vi "gesture.vi"() -> ()   [LabVIEW 2012]
uses:
  <vilib>/University of Leeds/Kinesthesia Toolkit for Microsoft Kinect/_Polymorphic Configure/Event-Skeleton.vi
  <vilib>/University of Leeds/Kinesthesia Toolkit for Microsoft Kinect/_Polymorphic Close/Close-Skeleton.vi
  <vilib>/University of Leeds/Kinesthesia Toolkit for Microsoft Kinect/_Polymorphic Read/Read-Skeleton.vi
panel:
  in  "文件路径（使用对话框）":path=path "E:/djangowork/ni/main/status.txt"
  out "连接的字符串":string
  in  "Target":string="dstp://localhost/para" caption="目标"
  out "量表":dbl(knob) scale=-180.0..180.0
  out "转动状态标识":u8
  out "待转度数":dbl
  out "state":u8
  out "缩放手势识别":bool
  out "放大杆":dbl(slide) scale=0.5..1000.0
  in  "左手z数组":dbl[](array[numeric])
  in  "右手z数组":dbl[](array[numeric])
  out "缩放手势计数":u8
  in  "下限":dbl
  in  "上限":dbl=0.2
  in  "左肩y数组":dbl[](array[numeric])
  in  "右手y数组":dbl[](array[numeric])
  in  "右划阈值":dbl=0.08
  in  "左划阈值":dbl=-0.08
  in  "右上下阈值":dbl=0.2
  out "右挥手势判断":bool
  in  "左上下阈值":dbl=0.2
  in  "右手x数组":dbl[](array[numeric])
  in  "左手y数组":dbl[](array[numeric])
  out "左挥手势判断":bool
  in  "数组索引":i32
  in  "左手x数组":dbl[](array[numeric])
  in  "布尔":bool
  out "error out":errorcluster
  in  "error in (no error)":errorcluster
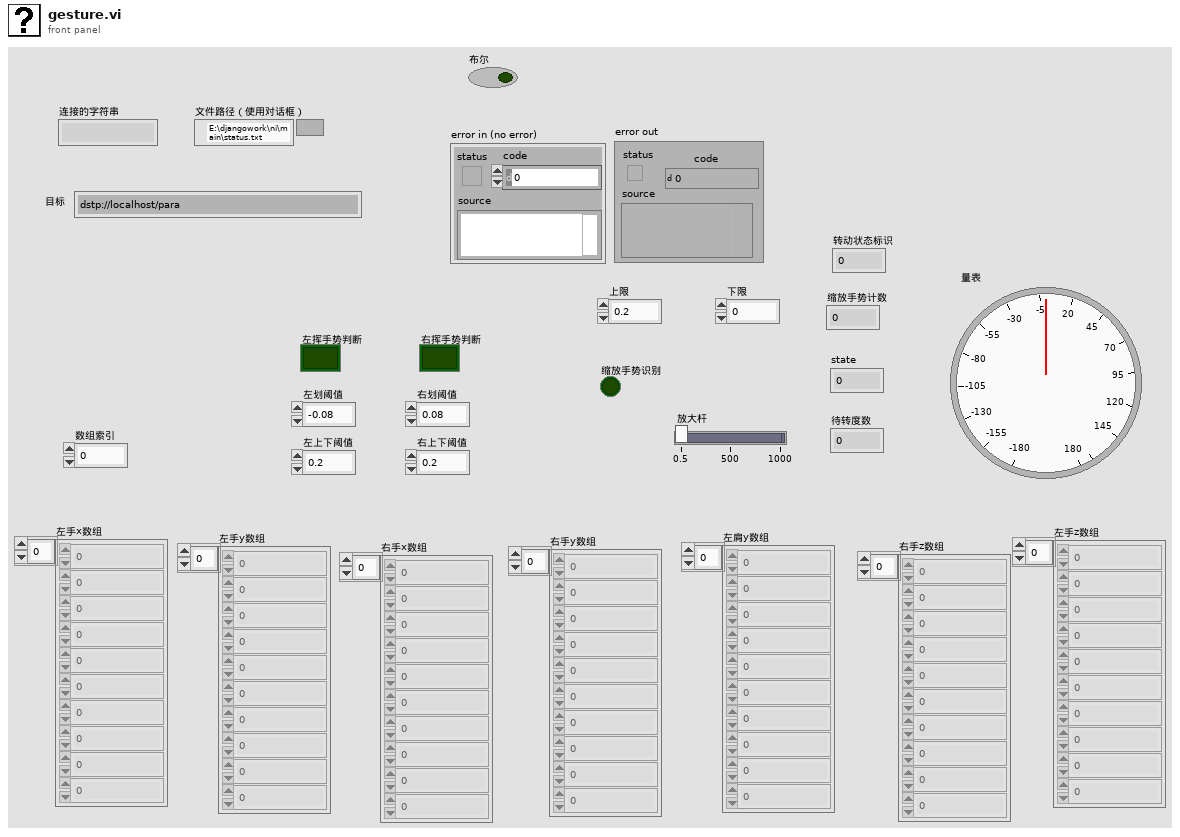
[diagram p1: front panel]
types:
  T1 = cluster{cluster{"reference out":refnum<k24>, "KinectSensors":refnum<k24>}, "get_Item":refnum<k24>}
  T2 = cluster{"reference out":refnum<k24>, "KinectSensors":refnum<k24>, "SkeletonStream":refnum<k24>, refnum<k24>[], "get_Item":refnum<k24>}
  T3 = enum16{"hip centre", "spine", "shoulder centre", "head", "shoulder left", "elbow left", "wrist left", "hand left", "shoulder right", "elbow right", "wrist right", "hand right", "hip left", "knee left", "ankle left", "foot left", "hip right", "knee right", "ankle right", "foot right"}
  T4 = enum16{"open", "replace", "create", "open or create", "replace or create", "replace or create with confirmation"}
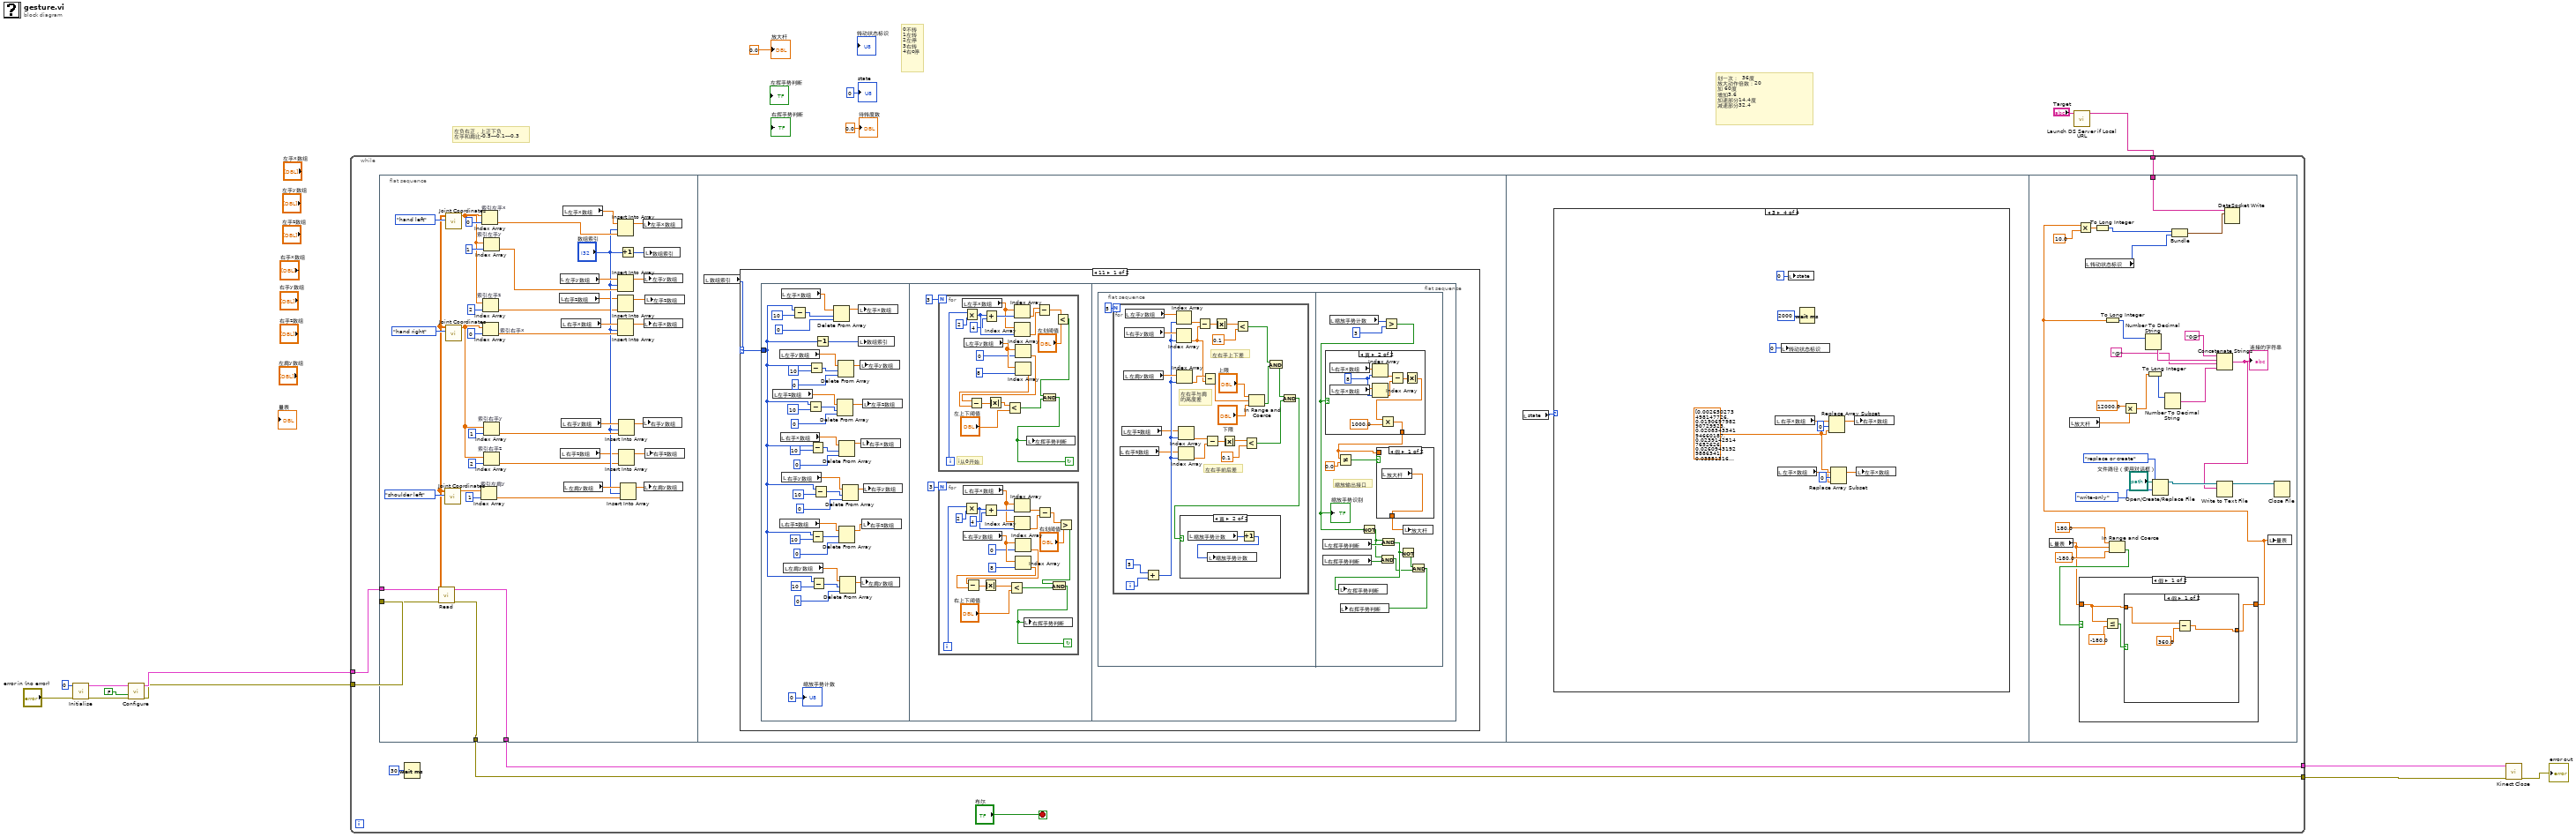
[diagram p0: block diagram]
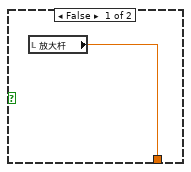
[diagram p4: hidden frame]
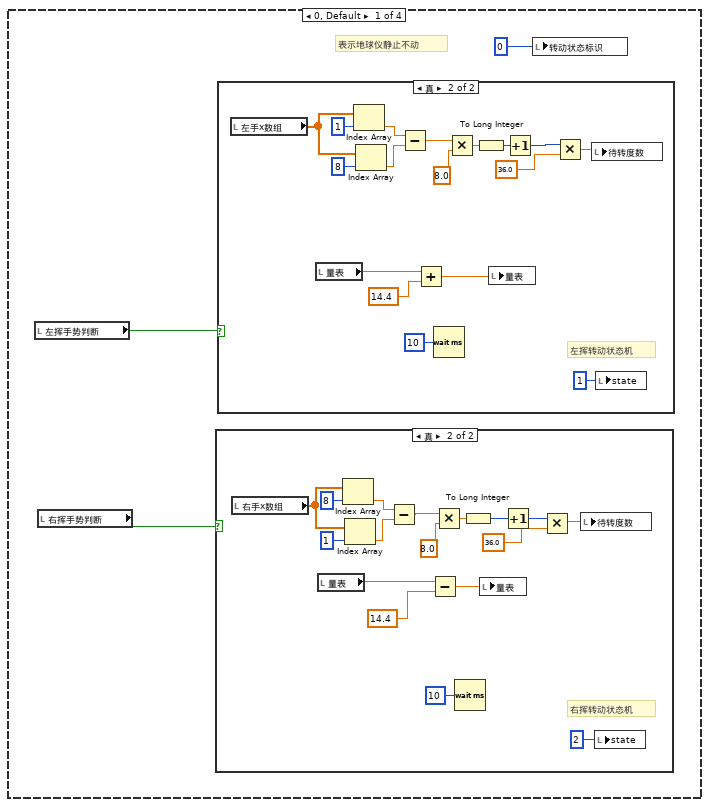
[diagram p6: hidden frame]
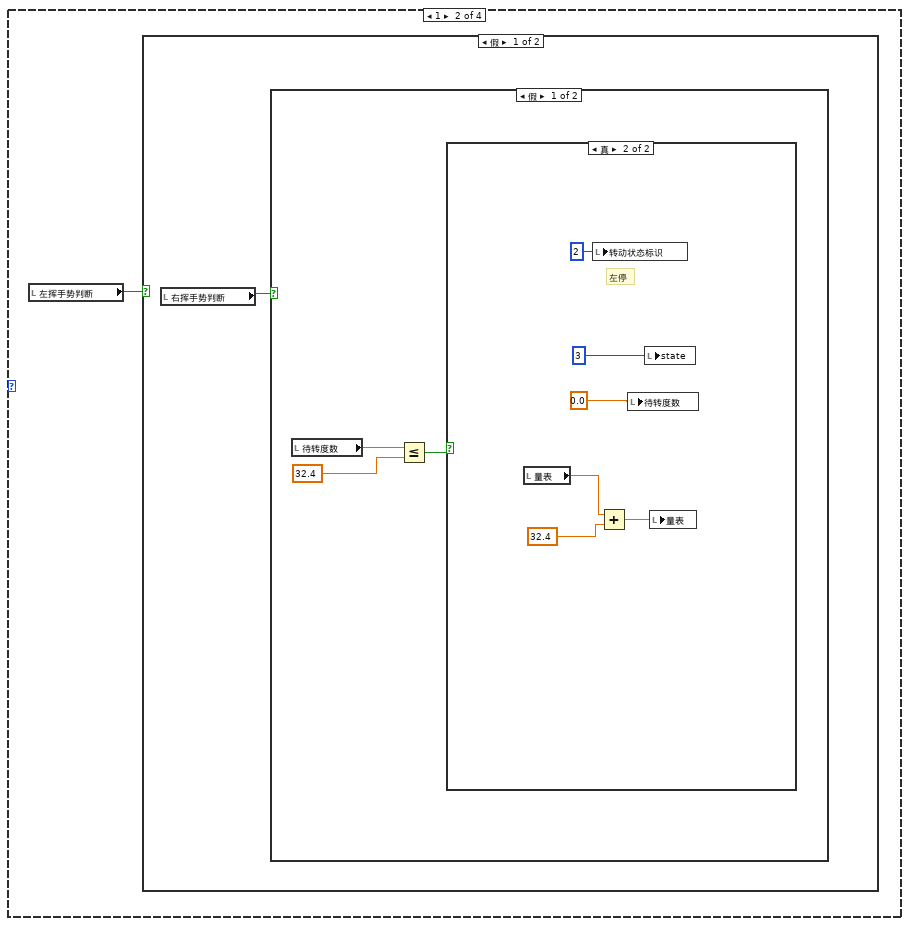
[diagram p9: hidden frame]
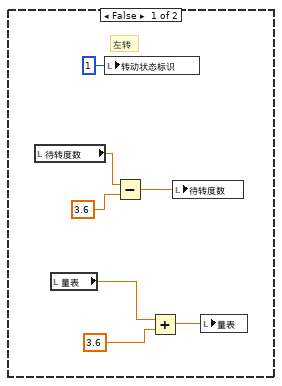
[diagram p10: hidden frame]
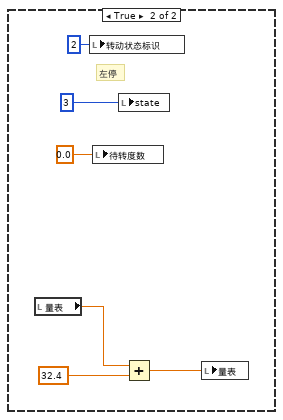
[diagram p11: hidden frame]
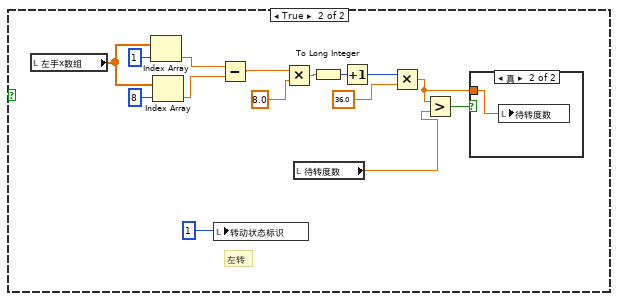
[diagram p12: hidden frame]
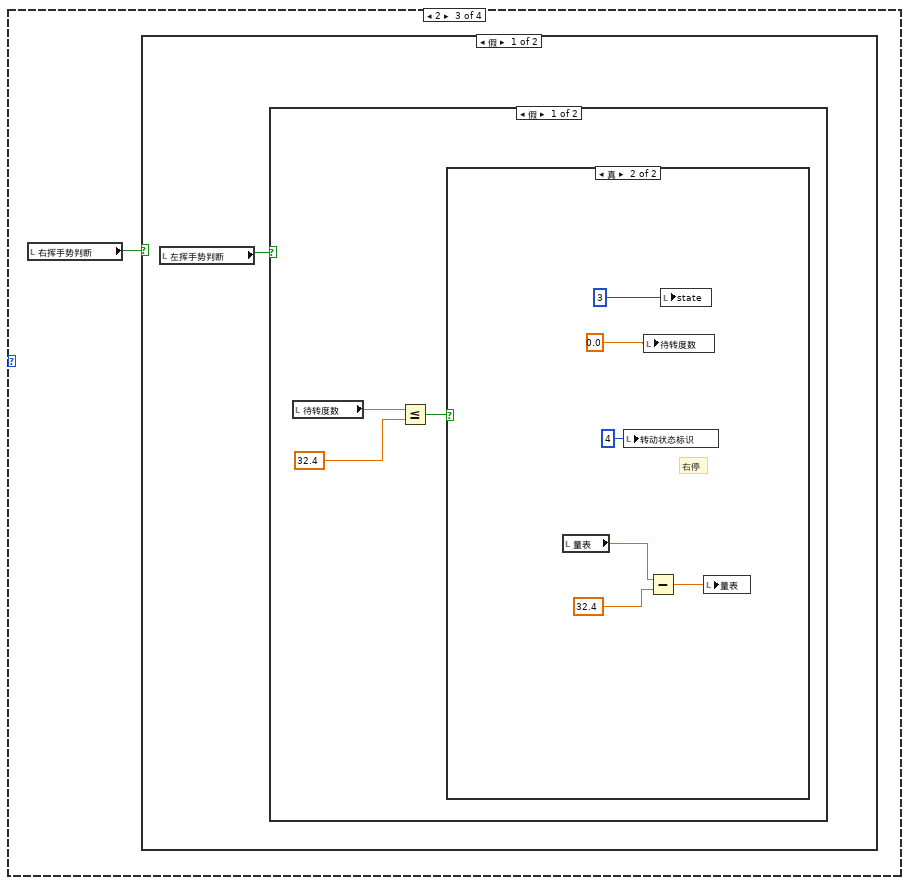
[diagram p14: hidden frame]
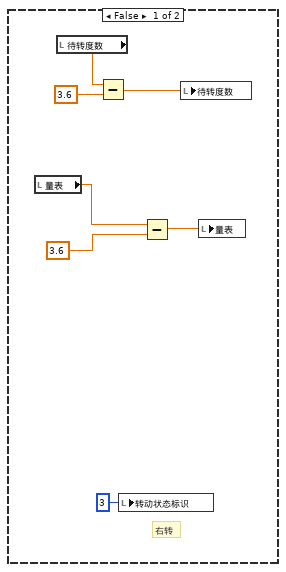
[diagram p15: hidden frame]
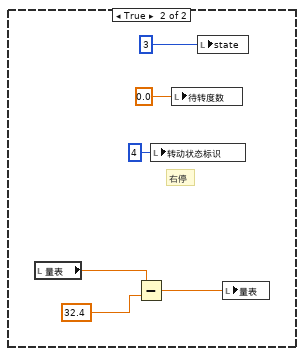
[diagram p16: hidden frame]
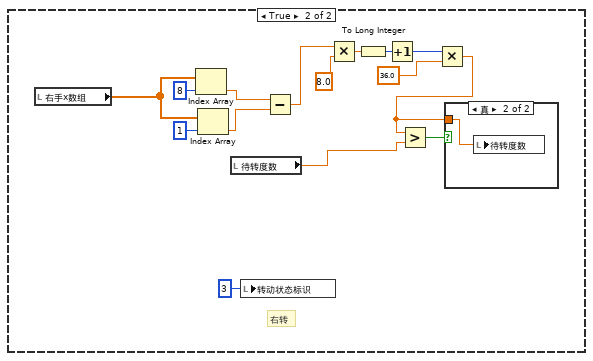
[diagram p17: hidden frame]
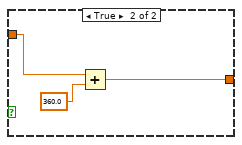
[diagram p19: hidden frame]
diagram:
  # "划一次：  36度\n放大动作倍数：20\n加 60度\n增加3.6\n加速部分14.4度\n减速部分32.4"
  # "0不转\n1左转\n2左停\n3右转\n4右c停"
  # "左负右正，上正下负\n左手和肩比-0.5---0.1---0.3"
  n1 = call <vilib>:"Initialise.vi"("Kinect Number"=0, "error in (no error)"="error in (no error)") -> ("Kinect References out"=w11:T1, "error out"=w14:errorcluster)  [unwired: 12 in]
  n2 = call-poly <vilib>:"Configure.vi"("Kinect References in"=w11, "Skeleton Smoothing"=FALSE, "error in"=w14) -> ("Kinect References out"=w10:T2, "error out"=w9:errorcluster)  [unwired: 11 in]
  n3 = call <vilib>:"Launch DS Server if Local URL.vi"("URL"="Target") -> ("Duplicate URL"=w2:string)  [unwired: 1 in, 5 out]
  n4 = while {
    tunnel: w10 -> [w20]
    tunnel: w9 -> [w21]
    tunnel: [w19] -> w8
    tunnel: [w18] -> w7
    tunnel: w2 -> [w16]
    stop <- "布尔" stop-if-true
    n5 = flat-sequence {
      tunnel: w21 -> [w63]
      tunnel: w20 -> [w62]
      tunnel: [w61] -> w19
      tunnel: [w60] -> w18
      tunnel: w16 -> [w339]
      frame #0 {
        n6 = call-poly <vilib>:"Read.vi"("Kinect References in"=w62, "error in (no error)"=w63) -> ("Primary Skeleton Array"=w37:dbl[][], "Kinect References out"=w61:T2, "error out"=w60:errorcluster)  [unwired: 10 in, 1 out]
        n7 = call <vilib>:"Joint Coordinates.vi"("Joint 1"=T3."shoulder left", "Array of Joint Positions"=w37) -> ("Joint Coordinates"=w38:dbl[])  [unwired: 8 in, 1 out]
        n8 = call <vilib>:"Joint Coordinates.vi"("Joint 1"=T3."hand left", "Array of Joint Positions"=w37) -> ("Joint Coordinates"=w28:dbl[])  [unwired: 8 in, 1 out]
        n9 = call <vilib>:"Joint Coordinates.vi"("Joint 1"=T3."hand right", "Array of Joint Positions"=w37) -> ("Joint Coordinates"=w27:dbl[])  [unwired: 8 in, 1 out]
        n10 = Index Array "索引左肩y"(array=w38, index=1 ("索引")) -> (element=w36:dbl)
        n11 = Index Array "索引左手x"(array=w28, index=0 ("索引")) -> (element=w56:dbl)
        n12 = Index Array "索引左手z"(array=w28, index=2 ("索引")) -> (element=w29:dbl)
        n13 = Index Array "索引右手x"(array=w27, index=0 ("索引")) -> (element=w47:dbl)
        n14 = Index Array "索引左手y"(array=w28, index=1 ("索引")) -> (element=w52:dbl)
        n15 = Index Array "索引右手y"(array=w27, index=1 ("索引")) -> (element=w43:dbl)
        n16 = Index Array "索引右手z"(array=w27, index=2 ("索引")) -> (element=w31:dbl)
        n17 = local read "右手z数组"() -> (w26:dbl[])
        n18 = local read "左手y数组"() -> (w51:dbl[])
        n19 = local read "右手z数组"() -> (w23:dbl[])
        n20 = local read "右手x数组"() -> (w46:dbl[])
        n21 = local read "右手y数组"() -> (w41:dbl[])
        n22 = local read "左手x数组"() -> (w55:dbl[])
        n23 = local read "左肩y数组"() -> (w35:dbl[])
        n24 = Insert Into Array(array=w55, index="数组索引", new element=w56) -> (w54:dbl[])
        n25 = Insert Into Array(array=w51, index="数组索引", new element=w52) -> (w50:dbl[])
        n26 = Insert Into Array(array=w26, new element=w29) -> (w25:dbl[])  [unwired: 1 in]
        n27 = Insert Into Array(array=w46, index="数组索引", new element=w47) -> (w45:dbl[])
        n28 = Insert Into Array(array=w41, index="数组索引", new element=w43) -> (w42:dbl[])
        n29 = Insert Into Array(array=w23, new element=w31) -> (w24:dbl[])  [unwired: 1 in]
        n30 = Increment(x="数组索引") -> (x+1=w53:i32)
        n31 = Insert Into Array(array=w35, index="数组索引", new element=w36) -> (w34:dbl[])
        n32 = local write "左手x数组"(w54) -> ()
        n33 = local write "右手y数组"(w42) -> ()
        n34 = local write "左手y数组"(w50) -> ()
        n35 = local write "右手x数组"(w45) -> ()
        n36 = local write "左肩y数组"(w34) -> ()
        n37 = local write "数组索引"(w53) -> ()
        n38 = local write "右手z数组"(w24) -> ()
        n39 = local write "左手z数组"(w25) -> ()
      }
      frame #1 {
        n40 = local read "数组索引"() -> (w64:i32)
        n41 = case shown="11" w64 {
          selector: w64 -> [w65 _]
          frame 11 {
            n42 = flat-sequence {
              tunnel: w65 -> [w66]
              frame #0 {
                n43 = local read "左手z数组"() -> (w70:dbl[])
                n44 = local read "左手y数组"() -> (w91:dbl[])
                n45 = local read "右手z数组"() -> (w67:dbl[])
                n46 = local read "右手x数组"() -> (w90:dbl[])
                n47 = local read "左手x数组"() -> (w102:dbl[])
                n48 = local read "右手y数组"() -> (w84:dbl[])
                n49 = local read "左肩y数组"() -> (w79:dbl[])
                n50 = Subtract(x=w66, y=10) -> (x-y=w99:i32)
                n51 = Subtract(x=w66, y=10) -> (x-y=w72:i32)
                n52 = Subtract(x=w66, y=10) -> (x-y=w95:i32)
                n53 = Subtract(x=w66, y=10) -> (x-y=w92:i32)
                n54 = Subtract(x=w66, y=10) -> (x-y=w75:i32)
                n55 = Subtract(x=w66, y=10) -> (x-y=w81:i32)
                n56 = Subtract(x=w66, y=10) -> (x-y=w86:i32)
                n57 = Decrement(x=w66) -> (x-1=w98:i32)
                n58 = Delete From Array(array=w102, length=w99, index=0 ("索引")) -> (array with subset deleted=w101:dbl[])  [unwired: 1 out]
                n59 = Delete From Array(array=w70, length=w72, index=0 ("索引")) -> (array with subset deleted=w69:dbl[])  [unwired: 1 out]
                n60 = Delete From Array(array=w91, length=w95, index=0 ("索引")) -> (array with subset deleted=w89:dbl[])  [unwired: 1 out]
                n61 = Delete From Array(array=w90, length=w92, index=0 ("索引")) -> (array with subset deleted=w88:dbl[])  [unwired: 1 out]
                n62 = Delete From Array(array=w67, length=w75, index=0 ("索引")) -> (array with subset deleted=w68:dbl[])  [unwired: 1 out]
                n63 = Delete From Array(array=w79, length=w81, index=0 ("索引")) -> (array with subset deleted=w78:dbl[])  [unwired: 1 out]
                n64 = Delete From Array(array=w84, length=w86, index=0 ("索引")) -> (array with subset deleted=w83:dbl[])  [unwired: 1 out]
                n65 = local write "左手x数组"(w101) -> ()
                n66 = local write "数组索引"(w98) -> ()
                n67 = local write "左手y数组"(w89) -> ()
                n68 = local write "左肩y数组"(w78) -> ()
                n69 = local write "右手x数组"(w88) -> ()
                n70 = local write "右手z数组"(w68) -> ()
                n71 = local write "左手z数组"(w69) -> ()
                n72 = local write "右手y数组"(w83) -> ()
                "缩放手势计数" <- u8 0 ("放大判断计数")
              }
              frame #1 {
                n73 = for {
                  N: 3 -> [_]
                  i -> [w142]
                  stop <- w134 continue-if-true
                  # "i从0开始"
                  n74 = local read "左手x数组"() -> (w145:dbl[])
                  n75 = local read "左手y数组"() -> (w133:dbl[])
                  n76 = Multiply(x=w142, y=2) -> (x*y=w144:i32)
                  n77 = Add(x=w144, y=4) -> (x+y=w146:i32)
                  n78 = Index Array(array=w145, index=w146) -> (element=w132:dbl)
                  n79 = Index Array(array=w145, index=w144) -> (element=w131:dbl)
                  n80 = Index Array(array=w133, index=0 ("索引")) -> (element=w141:dbl)
                  n81 = Index Array(array=w133, index=8 ("索引")) -> (element=w140:dbl)
                  n82 = Subtract(x=w141, y=w140) -> (x-y=w139:dbl)
                  n83 = Absolute Value(x=w139) -> (abs(x)=w138:dbl)
                  n84 = Less?(x=w138, y="左上下阈值") -> (x < y?=w135:bool)
                  n85 = Subtract(x=w132, y=w131) -> (x-y=w130:dbl)
                  n86 = Less?(x=w130, y="左划阈值") -> (x < y?=w136:bool)
                  n87 = And(x=w136, y=w135) -> (x .and. y?=w134:bool)
                  n88 = local write "左挥手势判断"(w134) -> ()
                }
                n89 = for {
                  N: 3 -> [_]
                  i -> [w122]
                  stop <- w111 continue-if-true
                  n90 = local read "右手y数组"() -> (w120:dbl[])
                  n91 = local read "右手x数组"() -> (w121:dbl[])
                  n92 = Multiply(x=w122, y=2) -> (x*y=w123:i32)
                  n93 = Add(x=w123, y=4) -> (x+y=w124:i32)
                  n94 = Index Array(array=w121, index=w124) -> (element=w119:dbl)
                  n95 = Index Array(array=w121, index=w123) -> (element=w118:dbl)
                  n96 = Index Array(array=w120, index=0 ("索引")) -> (element=w117:dbl)
                  n97 = Index Array(array=w120, index=8 ("索引")) -> (element=w116:dbl)
                  n98 = Subtract(x=w117, y=w116) -> (x-y=w115:dbl)
                  n99 = Absolute Value(x=w115) -> (abs(x)=w113:dbl)
                  n100 = Less?(x=w113, y="右上下阈值") -> (x < y?=w112:bool)
                  n101 = Subtract(x=w119, y=w118) -> (x-y=w110:dbl)
                  n102 = Greater?(x=w110, y="右划阈值") -> (0:w109:bool)
                  n103 = And(x=w109, y=w112) -> (x .and. y?=w111:bool)
                  n104 = local write "右挥手势判断"(w111) -> ()
                }
              }
              frame #2 {
                n105 = flat-sequence {
                  frame #0 {
                    n106 = for {
                      N: 5 -> [_]
                      i -> [w161]
                      # "左右手上下差"
                      # "左右手前后差"
                      # "左右手与肩\n的高度差"
                      n107 = local read "右手z数组"() -> (w157:dbl[])
                      n108 = local read "左手z数组"() -> (w158:dbl[])
                      n109 = local read "左肩y数组"() -> (w170:dbl[])
                      n110 = local read "右手y数组"() -> (w174:dbl[])
                      n111 = local read "左手y数组"() -> (w175:dbl[])
                      n112 = Add(x=5, y=w161) -> (x+y=w159:i32)
                      n113 = Index Array(array=w175, index=w159) -> (element=w173:dbl)
                      n114 = Index Array(array=w174, index=w159) -> (element=w168:dbl)
                      n115 = Index Array(array=w170, index=w159) -> (element=w169:dbl)
                      n116 = Index Array(array=w158, index=w159) -> (element=w155:dbl)
                      n117 = Index Array(array=w157, index=w159) -> (element=w154:dbl)
                      n118 = Subtract(x=w173, y=w168) -> (x-y=w162:dbl)
                      n119 = Subtract(x=w169, y=w168) -> (x-y=w165:dbl)
                      n120 = Subtract(x=w155, y=w154) -> (x-y=w156:dbl)
                      n121 = Absolute Value(x=w162) -> (abs(x)=w172:dbl)
                      n122 = Absolute Value(x=w156) -> (abs(x)=w153:dbl)
                      n123 = Less?(x=w172, y=0.1 ("左右手上下差")) -> (x < y?=w163:bool)
                      n124 = Less?(x=w153, y=0.1 ("左右手前后差")) -> (x < y?=w151:bool)
                      n125 = In Range and Coerce(upper limit="上限", x=w165, lower limit="下限") -> (In Range?=w164:bool)  [unwired: 1 out]
                      n126 = And(x=w163, y=w164) -> (x .and. y?=w152:bool)
                      n127 = And(x=w152, y=w151) -> (x .and. y?=w150:bool)
                      n128 = case shown="真" w150 {
                        frame False {
                        }
                        frame True {
                          n129 = local read "缩放手势计数"() -> (w177:u8)
                          n130 = Increment(x=w177) -> (x+1=w176:u8)
                          n131 = local write "缩放手势计数"(w176) -> ()
                        }
                      }
                    }
                  }
                  frame #1 {
                    # "缩放输出接口"
                    n132 = local read "左挥手势判断"() -> (w188:bool)
                    n133 = local read "右挥手势判断"() -> (w186:bool)
                    n134 = local read "缩放手势计数"() -> (w191:u8)
                    n135 = Greater?(x=w191, y=u8 3) -> (0:w182:bool)
                    "缩放手势识别" <- w182
                    n136 = case shown="真" w182 {
                      tunnel: [w194 w197] -> w179
                      frame False {
                        n137 = local read "放大杆"() -> (w194:dbl)
                      }
                      frame True {
                        w195 = 8 ("索引")
                        n138 = local read "右手x数组"() -> (w202:dbl[])
                        n139 = local read "左手x数组"() -> (w203:dbl[])
                        n140 = Index Array(array=w202, index=w195) -> (element=w200:dbl)
                        n141 = Index Array(array=w203, index=w195) -> (element=w199:dbl)
                        n142 = Subtract(x=w200, y=w199) -> (x-y=w201:dbl)
                        n143 = Absolute Value(x=w201) -> (abs(x)=w198:dbl)
                        n144 = Multiply(x=w198, y=1000.0 ("调整")) -> (x*y=w197:dbl)
                      }
                    }
                    n145 = Not Equal?(x=w179, y=0.0) -> (x != y?=w181:bool)
                    n146 = Not(x=w182) -> (.not. x?=w187:bool)
                    n147 = case shown="假" w181 {
                      tunnel: w179 -> [_ w193]
                      tunnel: [w192 w193] -> w178
                      frame False {
                        n148 = local read "放大杆"() -> (w192:dbl)
                      }
                      frame True {
                      }
                    }
                    n149 = And(x=w187, y=w186) -> (x .and. y?=w184:bool)
                    n150 = And(x=w187, y=w188) -> (x .and. y?=w189:bool)
                    n151 = local write "左挥手势判断"(w189) -> ()
                    n152 = Not(x=w189) -> (.not. x?=w185:bool)
                    n153 = local write "放大杆"(w178) -> ()
                    n154 = And(x=w185, y=w184) -> (x .and. y?=w183:bool)
                    n155 = local write "右挥手势判断"(w183) -> ()
                  }
                }
              }
            }
          }
          frame 0..10, Default {
          }
        }
      }
      frame #2 {
        n156 = local read "state"() -> (w204:u8)
        n157 = case shown="3" w204 {
          frame 0, Default {
            # "表示地球仪静止不动"
            n158 = local read "左挥手势判断"() -> (w207:bool)
            n159 = local read "右挥手势判断"() -> (w206:bool)
            n160 = case shown="真" w206 {
              frame False {
              }
              frame True {
                # "右挥转动状态机"
                n161 = local read "右手x数组"() -> (w219:dbl[])
                n162 = local read "量表"() -> (w215:dbl)
                n163 = Index Array(array=w219, index=8 ("索引")) -> (element=w220:dbl)
                n164 = Index Array(array=w219, index=1 ("索引")) -> (element=w221:dbl)
                n165 = Subtract(x=w220, y=w221) -> (x-y=w209:dbl)
                n166 = Subtract(x=w215, y=14.4) -> (x-y=w216:dbl)
                n167 = Multiply(x=w209, y=8.0) -> (x*y=w212:dbl)
                n168 = Wait (ms)(milliseconds to wait=u32 10 ("等待时间（毫秒）")) -> ()  [unwired: 1 out]
                n169 = To Long Integer(number=w212) -> (32bit integer=w211:i32)
                n170 = local write "量表"(w216) -> ()
                n171 = Increment(x=w211) -> (x+1=w210:i32)
                n172 = Multiply(x=w210, y=36.0) -> (x*y=w208:dbl)
                n173 = local write "待转度数"(w208) -> ()
                n174 = local write "state"(u8 2 ("state")) -> ()
              }
            }
            n175 = case shown="真" w207 {
              frame False {
              }
              frame True {
                # "左挥转动状态机"
                n176 = local read "左手x数组"() -> (w240:dbl[])
                n177 = local read "量表"() -> (w231:dbl)
                n178 = Index Array(array=w240, index=1 ("索引")) -> (element=w236:dbl)
                n179 = Index Array(array=w240, index=8 ("索引")) -> (element=w237:dbl)
                n180 = Subtract(x=w236, y=w237) -> (x-y=w235:dbl)
                n181 = Add(x=w231, y=14.4) -> (x+y=w229:dbl)
                n182 = Wait (ms)(milliseconds to wait=u32 10 ("等待时间（毫秒）")) -> ()  [unwired: 1 out]
                n183 = Multiply(x=w235, y=8.0) -> (x*y=w227:dbl)
                n184 = To Long Integer(number=w227) -> (32bit integer=w226:i32)
                n185 = local write "量表"(w229) -> ()
                n186 = Increment(x=w226) -> (x+1=w225:i32)
                n187 = Multiply(x=w225, y=36.0) -> (x*y=w232:dbl)
                n188 = local write "待转度数"(w232) -> ()
                n189 = local write "state"(u8 1 ("state")) -> ()
              }
            }
            n190 = local write "转动状态标识"(u8 0 ("转动状态标识")) -> ()
          }
          frame 1 {
            n191 = local read "左挥手势判断"() -> (w242:bool)
            n192 = case shown="假" w242 {
              frame False {
                n193 = local read "右挥手势判断"() -> (w243:bool)
                n194 = case shown="假" w243 {
                  frame False {
                    n195 = local read "待转度数"() -> (w246:dbl)
                    n196 = Less Or Equal?(x=w246, y=32.4) -> (x <= y?=w244:bool)
                    n197 = case shown="真" w244 {
                      frame False {
                        # "左转"
                        n198 = local read "待转度数"() -> (w253:dbl)
                        n199 = local read "量表"() -> (w250:dbl)
                        n200 = local write "转动状态标识"(u8 1 ("转动状态标识")) -> ()
                        n201 = Subtract(x=w253, y=3.6) -> (x-y=w251:dbl)
                        n202 = Add(x=w250, y=3.6) -> (x+y=w247:dbl)
                        n203 = local write "待转度数"(w251) -> ()
                        n204 = local write "量表"(w247) -> ()
                      }
                      frame True {
                        # "左停"
                        n205 = local read "量表"() -> (w255:dbl)
                        n206 = local write "转动状态标识"(u8 2 ("转动状态标识")) -> ()
                        n207 = Add(x=w255, y=32.4) -> (x+y=w254:dbl)
                        n208 = local write "待转度数"(0.0 ("待转多少度")) -> ()
                        n209 = local write "state"(u8 3 ("state")) -> ()
                        n210 = local write "量表"(w254) -> ()
                      }
                    }
                  }
                  frame True {
                    # "左停"
                    n211 = local read "量表"() -> (w261:dbl)
                    n212 = local write "转动状态标识"(u8 2 ("转动状态标识")) -> ()
                    n213 = local write "待转度数"(0.0 ("待转多少度")) -> ()
                    n214 = local write "state"(u8 3 ("state")) -> ()
                    n215 = Add(x=w261, y=32.4) -> (x+y=w260:dbl)
                    n216 = local write "量表"(w260) -> ()
                  }
                }
              }
              frame True {
                # "左转"
                n217 = local read "左手x数组"() -> (w276:dbl[])
                n218 = Index Array(array=w276, index=1 ("索引")) -> (element=w277:dbl)
                n219 = Index Array(array=w276, index=8 ("索引")) -> (element=w278:dbl)
                n220 = local write "转动状态标识"(u8 1 ("转动状态标识")) -> ()
                n221 = Subtract(x=w277, y=w278) -> (x-y=w267:dbl)
                n222 = Multiply(x=w267, y=8.0) -> (x*y=w270:dbl)
                n223 = local read "待转度数"() -> (w275:dbl)
                n224 = To Long Integer(number=w270) -> (32bit integer=w269:i32)
                n225 = Increment(x=w269) -> (x+1=w268:i32)
                n226 = Multiply(x=w268, y=36.0) -> (x*y=w266:dbl)
                n227 = Greater?(x=w266, y=w275) -> (0:w274:bool)
                n228 = case shown="真" w274 {
                  tunnel: w266 -> [_ w281]
                  frame False {
                  }
                  frame True {
                    n229 = local write "待转度数"(w281) -> ()
                  }
                }
              }
            }
          }
          frame 2 {
            n230 = local read "右挥手势判断"() -> (w282:bool)
            n231 = case shown="假" w282 {
              frame False {
                n232 = local read "左挥手势判断"() -> (w283:bool)
                n233 = case shown="假" w283 {
                  frame False {
                    n234 = local read "待转度数"() -> (w286:dbl)
                    n235 = Less Or Equal?(x=w286, y=32.4) -> (x <= y?=w284:bool)
                    n236 = case shown="真" w284 {
                      frame False {
                        # "右转"
                        n237 = local read "量表"() -> (w290:dbl)
                        n238 = local read "待转度数"() -> (w293:dbl)
                        n239 = Subtract(x=w293, y=3.6) -> (x-y=w291:dbl)
                        n240 = local write "转动状态标识"(u8 3 ("转动状态标识")) -> ()
                        n241 = Subtract(x=w290, y=3.6) -> (x-y=w287:dbl)
                        n242 = local write "待转度数"(w291) -> ()
                        n243 = local write "量表"(w287) -> ()
                      }
                      frame True {
                        # "右停"
                        n244 = local read "量表"() -> (w295:dbl)
                        n245 = local write "转动状态标识"(u8 4 ("转动状态标识")) -> ()
                        n246 = local write "待转度数"(0.0 ("待转多少度")) -> ()
                        n247 = Subtract(x=w295, y=32.4) -> (x-y=w294:dbl)
                        n248 = local write "state"(u8 3 ("state")) -> ()
                        n249 = local write "量表"(w294) -> ()
                      }
                    }
                  }
                  frame True {
                    # "右停"
                    n250 = local read "量表"() -> (w301:dbl)
                    n251 = Subtract(x=w301, y=32.4) -> (x-y=w300:dbl)
                    n252 = local write "转动状态标识"(u8 4 ("转动状态标识")) -> ()
                    n253 = local write "待转度数"(0.0 ("待转多少度")) -> ()
                    n254 = local write "state"(u8 3 ("state")) -> ()
                    n255 = local write "量表"(w300) -> ()
                  }
                }
              }
              frame True {
                # "右转"
                n256 = local read "右手x数组"() -> (w316:dbl[])
                n257 = Index Array(array=w316, index=8 ("索引")) -> (element=w317:dbl)
                n258 = Index Array(array=w316, index=1 ("索引")) -> (element=w318:dbl)
                n259 = local read "待转度数"() -> (w315:dbl)
                n260 = local write "转动状态标识"(u8 3 ("转动状态标识")) -> ()
                n261 = Subtract(x=w317, y=w318) -> (x-y=w307:dbl)
                n262 = Multiply(x=w307, y=8.0) -> (x*y=w310:dbl)
                n263 = To Long Integer(number=w310) -> (32bit integer=w309:i32)
                n264 = Increment(x=w309) -> (x+1=w308:i32)
                n265 = Multiply(x=w308, y=36.0) -> (x*y=w306:dbl)
                n266 = Greater?(x=w306, y=w315) -> (0:w314:bool)
                n267 = case shown="真" w314 {
                  tunnel: w306 -> [_ w321]
                  frame False {
                  }
                  frame True {
                    n268 = local write "待转度数"(w321) -> ()
                  }
                }
              }
            }
          }
          frame 3 {
            w322 = dbl[] [0.002650273498147726, 0.019069798290729523, 0.020834334194660187, 0.02391425147652626, 0.02609431929886341, 0.03551316261291504, -0.021449454128742218, -0.018847979605197906, 0.018697425723075867, 0.06378649175167084] ("左肩y数组 2")
            n269 = local read "右手x数组"() -> (w323:dbl[])
            n270 = local read "左手x数组"() -> (w326:dbl[])
            n271 = local write "转动状态标识"(u8 0 ("转动状态标识")) -> ()
            n272 = local write "state"(u8 0 ("state")) -> ()
            n273 = Wait (ms)(milliseconds to wait=u32 2000 ("等待时间（毫秒）")) -> ()  [unwired: 1 out]
            n274 = Replace Array Subset(array=w323, new element=w322, index=0 ("索引")) -> (w324:dbl[])
            n275 = Replace Array Subset(array=w326, new element=w322, index=0 ("索引")) -> (w325:dbl[])
            n276 = local write "右手x数组"(w324) -> ()
            n277 = local write "左手x数组"(w325) -> ()
          }
        }
      }
      frame #3 {
        n278 = local read "量表"() -> (w354:dbl)
        n279 = local read "放大杆"() -> (w337:dbl)
        n280 = local read "转动状态标识"() -> (w338:u8)
        n281 = In Range and Coerce(upper limit=180.0 ("上限"), x=w354, lower limit=-180.0 ("下限")) -> (In Range?=w355:bool)  [unwired: 1 out]
        n282 = case shown="假" w355 {
          tunnel: w354 -> [w359 w368]
          tunnel: [w358 w368] -> w333
          frame False {
            n283 = Less Or Equal?(x=w359, y=-180.0) -> (x <= y?=w360:bool)
            n284 = case shown="假" w360 {
              tunnel: w359 -> [w364 w367]
              tunnel: [w362 w366] -> w358
              frame False {
                n285 = Subtract(x=w364, y=360.0) -> (x-y=w362:dbl)
              }
              frame True {
                n286 = Add(x=w367, y=360.0) -> (x+y=w366:dbl)
              }
            }
          }
          frame True {
          }
        }
        n287 = Multiply(x=w333, y=10.0) -> (x*y=w335:dbl)
        n288 = To Long Integer(number=w335) -> (32bit integer=w334:i32)
        n289 = To Long Integer(number=w333) -> (32bit integer=w332:i32)
        n290 = Multiply(x=12000.0, y=w337) -> (x*y=w341:dbl)
        n291 = Number To Decimal String(number=w332) -> (decimal integer string=w352:string)  [unwired: 1 in]
        n292 = To Long Integer(number=w341) -> (32bit integer=w348:i32)
        n293 = Open/Create/Replace File(file path (use dialog)="文件路径（使用对话框）", operation (0:open)=T4."replace or create" ("操作(0:open)"), access (0:read/write)=enum16{"read/write", "read-only", "write-only"}."write-only" ("权限(0:read/write)")) -> (refnum out=w346:refnum<file>)  [unwired: 3 in, 2 out]
        n294 = Number To Decimal String(number=w348) -> (decimal integer string=w349:string)  [unwired: 1 in]
        n295 = Bundle(w334, "转动状态标识"=w338) -> (w353:cluster{i32, "转动状态标识":u8})  [unwired: 1 in]
        n296 = Concatenate Strings("0@" ("字符串"), w352, "@" ("字符串"), w349) -> (w342:string)
        "连接的字符串" <- w342
        n297 = Write to Text File(file (use dialog)=w346, text=w342) -> (refnum out=w343:refnum<file>)  [unwired: 2 in, 2 out]
        n298 = DataSocket Write(10:w353, 11:w339) -> ()  [unwired: 2 in, 3 out]
        n299 = local write "量表"(w333) -> ()
        n300 = Close File(refnum=w343) -> ()  [unwired: 1 in, 2 out]
      }
    }
    n301 = Wait (ms)(milliseconds to wait=u32 30 ("等待时间（毫秒）")) -> ()  [unwired: 1 out]
  }
  n302 = call-poly <vilib>:"Kinect Close.vi"("Kinect References in"=w8, "error in"=w7) -> ("error out"=→"error out":errorcluster)  [unwired: 13 in]
  "state" <- u8 0 ("state")
  "待转度数" <- 0.0 ("待转多少度")
  "放大杆" <- 0.0 ("放大杆")
